vi "send move to stages.vi"(8 "error in (no error)":errorcluster, 11 "LineCCD in":refnum<class "LineCCD.lvclass">) -> (0 "error out":errorcluster, 3 "LineCCD out":refnum<class "LineCCD.lvclass">)   [LabVIEW 2012, in "LineCCD.lvclass"]
uses:
  LineCCD.lvclass
  <vilib>/Distrio/Murmex/GenericMessage/GenericMessage.lvclass
  <vilib>/Distrio/Murmex/Message/Message.lvclass
  <vilib>/Distrio/Murmex/Murmex/Murmex.lvclass
panel:
  in  "rel move to send":dbl[unit]
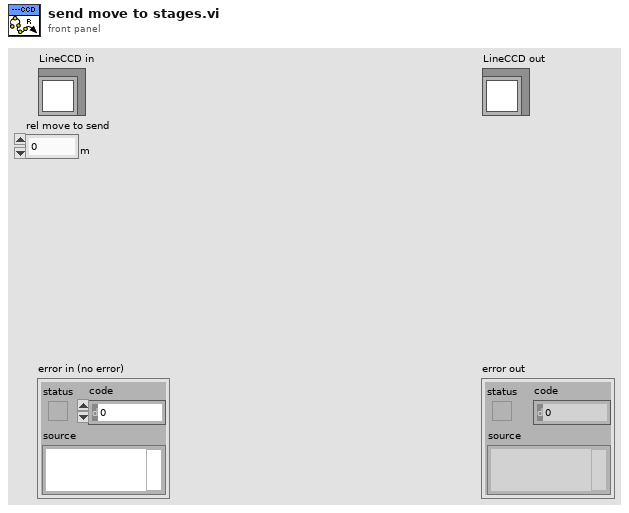
[diagram p1: front panel]
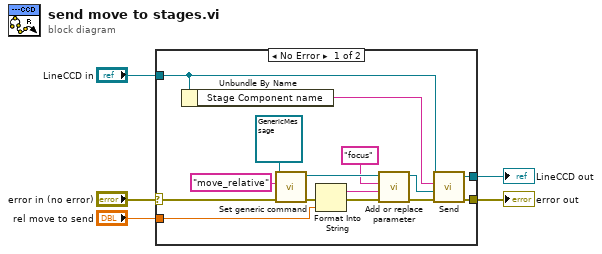
[diagram p0: block diagram]
diagram:
  n1 = case shown="No Error" "error in (no error)" {
    selector: "error in (no error)" -> [w11 w22]
    tunnel: [w10 w22] -> w4
    tunnel: [w6 w21] -> w2
    tunnel: "LineCCD in" -> [w7 w21]
    tunnel: "rel move to send" -> [w8 _]
    frame No Error {
      n2 = Unbundle By Name(w7) -> ("Stage Component name"=w9:string)
      n3 = call <vilib>:"Set generic command.vi"("error in (no error)"=w11, "generic command"="move_relative" ("command string"), "GenericMessage in"=refnum<class "GenericMessage.lvclass"> refnum ("Murmex.lvlib:GenericMessage")) -> ("error out"=w17:errorcluster, "GenericMessage out"=w20:refnum<class "GenericMessage.lvclass">)  [unwired: 7 in]
      n4 = Format Into String(error in=w17, w8) -> (resulting string=w15:string, error out=w16:errorcluster)  [unwired: 2 in]
      n5 = call <vilib>:"Add or replace parameter.vi"("error in (no error)"=w16, "value"=w15, "name"="focus", "Message in"=w20) -> ("error out"=w18:errorcluster, "Message out"=w19:refnum<class "GenericMessage.lvclass">)  [unwired: 6 in]
      n6 = call <vilib>:"Send.vi"("error in (no error)"=w18, "Message"=w19, "recipient"=w9, "Murmex in"=w7) -> ("error out"=w10:errorcluster, "Murmex out"=w6:refnum<class "LineCCD.lvclass">)  [unwired: 6 in]
    }
    frame Error {
    }
  }
  "error out" <- w4
  "LineCCD out" <- w2
